vi "LV70DateRecToTimeStamp.vi"(1 "date time rec":T2) -> (0 "Time Stamp":timestamp)   [LabVIEW 2020]
doc: "This VI replicates the behavior of prior versions of LabVIEW:\n1) date time rec does not have fractional seconds\n2) date time rec always represents local time\n3) On Windows and Macintosh opperating systems, date time rec is always in the appropriate DST (Daylight Saving) state\n\nFor future VI developement, the \"Date/Time To Seconds\" may be used in the new ways:\n1) date time rec may represent UTC time\n2) DST is used to calculate the appropriate time. For example:\n DST = 0 (Daylight Saving is off)\n date time rec is in Daylight Saving range\n Result time = date time rec time + Daylight Saving adjustment\nPass -1 for DST to avoid this conversion"
panel:
  in  "new date time rec":T1
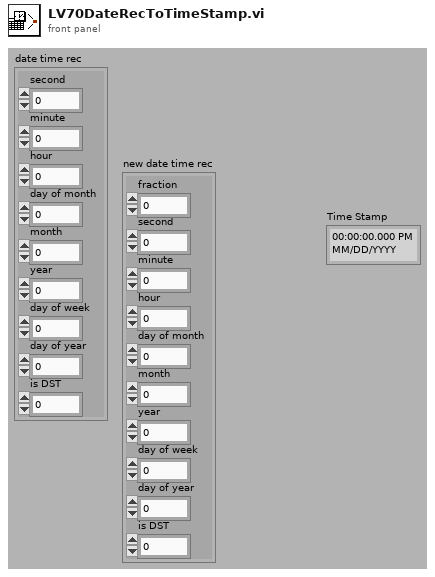
[diagram p1: front panel]
types:
  T1 = cluster{"fraction":dbl, "second":i32, "minute":i32, "hour":i32, "day of month":i32, "month":i32, "year":i32, "day of week":i32, "day of year":i32, "is DST":i32}
  T2 = cluster{"second":i32, "minute":i32, "hour":i32, "day of month":i32, "month":i32, "year":i32, "day of week":i32, "day of year":i32, "is DST":i32}
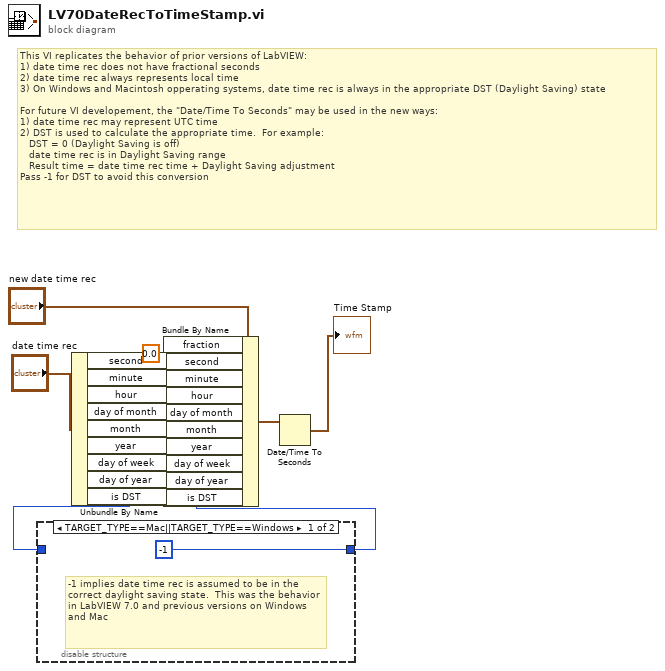
[diagram p0: block diagram]
diagram:
  # "This VI replicates the behavior of prior versions of LabVIEW:\n1) date time rec does not have fractional seconds\n2) date time rec always represents local time\n3) On Windows and Macintosh opperating systems, date time rec is always in the appropriate DST (Daylight Saving) state\n\nFor future VI developement, the \"Date/Time To Seconds\" may be used in the new ways:\n1) date time rec may represent UTC time\n2) DST is used to calculate the appropriate time.  For example:\n   DST = 0 (Daylight Saving is off)\n   date time rec is in Daylight Saving range\n   Result time = date time rec time + Daylight Saving adjustment\nPass -1 for DST to avoid this conversion"
  n1 = Unbundle By Name("date time rec") -> ("second"=w13:i32, "minute"=w12:i32, "hour"=w11:i32, "day of month"=w10:i32, "month"=w9:i32, "year"=w8:i32, "day of week"=w7:i32, "day of year"=w6:i32, "is DST"=w2:i32)
  n2 = disable-structure shown="TARGET_TYPE==Mac||TARGET_TYPE==Windows" {
    disable-tunnel: w2 -> [_ w17]
    disable-tunnel: [-1 ("is DST") w17] -> w1
    frame condition #0 (active) {
      # "-1 implies date time rec is assumed to be in the correct daylight saving state.  This was the behavior in LabVIEW 7.0 and previous versions on Windows and Mac"
    }
    frame condition #1 {
    }
  }
  n3 = Bundle By Name(cluster="new date time rec", "fraction"=0.0, "second"=w13, "minute"=w12, "hour"=w11, "day of month"=w10, "month"=w9, "year"=w8, "day of week"=w7, "day of year"=w6, "is DST"=w1) -> (w5:T1)
  n4 = Date/Time To Seconds(2:w5) -> (0:→"Time Stamp":timestamp)  [unwired: 1 in]
